vi "Update Actuator Data Timestamp.vi"(8 "error in (no error)":errorcluster, 11 "Model in":refnum<class "Model.lvclass">) -> (0 "error out":errorcluster, 3 "Model out":refnum<class "Model.lvclass">)   [LabVIEW 2016, in "Model.lvclass"]
uses:
  Model.lvclass
  Model.lvclass/Model.ctl
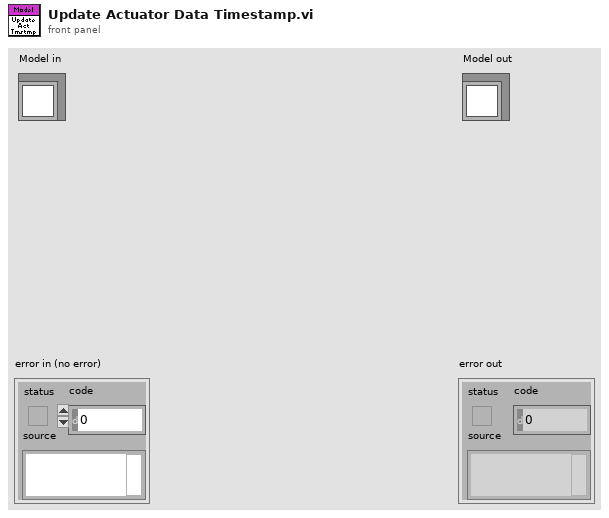
[diagram p1: front panel]
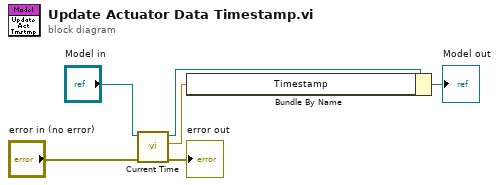
[diagram p0: block diagram]
diagram:
  n1 = call "Current Time.vi"("error in (no error)"="error in (no error)", "Model in"="Model in") -> ("error out"=→"error out":errorcluster, "Time"=w3:dbl, "Model out"=w4:refnum<class "Model.lvclass">)  [unwired: 7 in]
  n2 = Bundle By Name(cluster=w4, "Timestamp"=w3) -> (→"Model out":refnum<class "Model.lvclass">)
